vi "ContainsFile_WithFileNotIncluded_ReturnsFalse.vi"() -> ()   [LabVIEW 2017, in "WhitelistTest.lvlib"]
uses:
  WhitelistTest.lvlib
  Whitelist/Whitelist.lvclass
  Assertion/Assertion.lvlib
panel:
  out "error out":errorcluster
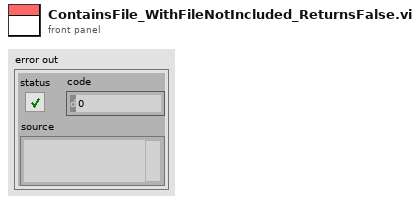
[diagram p1: front panel]
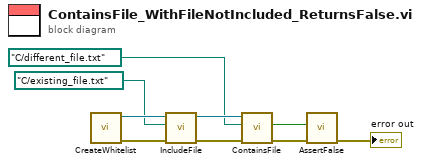
[diagram p0: block diagram]
diagram:
  n1 = call "CreateWhitelist.vi"() -> ("error out"=w9:errorcluster, "Whitelist out"=w7:refnum<class "Whitelist.lvclass">)  [unwired: 10 in]
  n2 = call "IncludeFile.vi"("error in (no error)"=w9, "Path"=path "C:/existing_file.txt", "Whitelist in"=w7) -> ("error out"=w8:errorcluster, "Whitelist out"=w6:refnum<class "Whitelist.lvclass">)  [unwired: 7 in]
  n3 = call "ContainsFile.vi"("error in (no error)"=w8, "Path"=path "C:/different_file.txt", "Whitelist in"=w6) -> ("error out"=w3:errorcluster, "Is Whitelisted?"=w4:bool)  [unwired: 6 in, 1 out]
  n4 = call "AssertFalse.vi"("error in (no error)"=w3, "Condition"=w4) -> ("error out"=→"error out":errorcluster)  [unwired: 9 in]
